vi "WebView_Init.vi"(8 "Error In":errorcluster, 11 "object in":refnum<class "WebView.lvclass">) -> (0 "Error Out":errorcluster, 3 "object out":refnum<class "WebView.lvclass">)   [LabVIEW 2024, in "WebView.lvclass"]
uses:
  WebView.lvclass
  WebView.lvclass/WebView.ctl
  <vilib>/sklein/WebView2/Libs/Microsoft.Web.WebView2.Core.dll
  Resources--cluster.ctl
  <vilib>/sklein/WebView2/Webview2 Control/Source Changed Event Data.ctl
  <vilib>/sklein/WebView2/Webview2 Control/WebView2 Control.xctl
  <vilib>/sklein/WebView2/Webview2 Control/Navigation Start Event Data.ctl
  <vilib>/sklein/WebView2/Webview2 Control/Navigation Event Data.ctl
  Events--cluster.ctl
  Navigation Event Data--cluster.ctl
  Source Changed Event Data--cluster.ctl
  Navigation Start Event Data--cluster.ctl
  <vilib>/sklein/WebView2/Libs/Microsoft.Web.WebView2.WinForms.dll
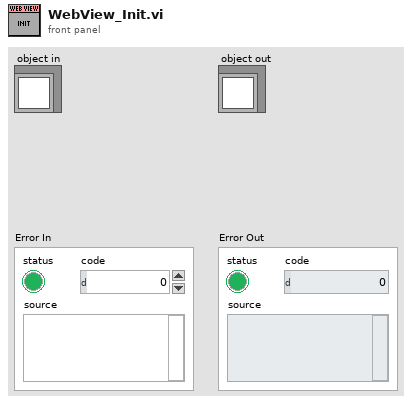
[diagram p1: front panel]
types:
  T1 = typedef "Navigation Start Event Data--cluster.ctl" = cluster{"AdditionalAllowedFrameAncestors":string, "Cancel":bool, "IsRedirected":bool, "IsUserInitiated":bool, "NavigationId":u64, "NavigationKind":i32, "RequestHeaders":refnum<k24>, "Uri":string}
  T2 = typedef "Navigation Event Data--cluster.ctl" = cluster{"HttpStatusCode":i32, "IsSuccess?":bool, "NavigationId":u64, "WebErrorStatus":i32}
  T3 = cluster{"Source":string, "WebMessageAsJson":string}
  T4 = typedef "WebView.lvclass/Events--cluster.ctl" = cluster{"Navigation Complete Event":refnum<user-event>, "Source Changed Event":refnum<user-event>, "Document Title Changed Event":refnum<user-event>, "Status Bar Text Changed":refnum<user-event>, "Web Message Received":refnum<user-event>, "Window Close Requested":refnum<user-event>, "DOM Loaded":refnum<user-event>, "Navigation Started Event":refnum<user-event>}
  T5 = typedef "Source Changed Event Data--cluster.ctl" = cluster{"Source":string, "IsNewDocument":bool}
  T6 = typedef "WebView.lvclass/Resources--cluster.ctl" = cluster{"WebView2":refnum<k24>, "Webview2 Core":refnum<k24>, "event callback":refnum<k27>, "Environment":refnum<k24>}
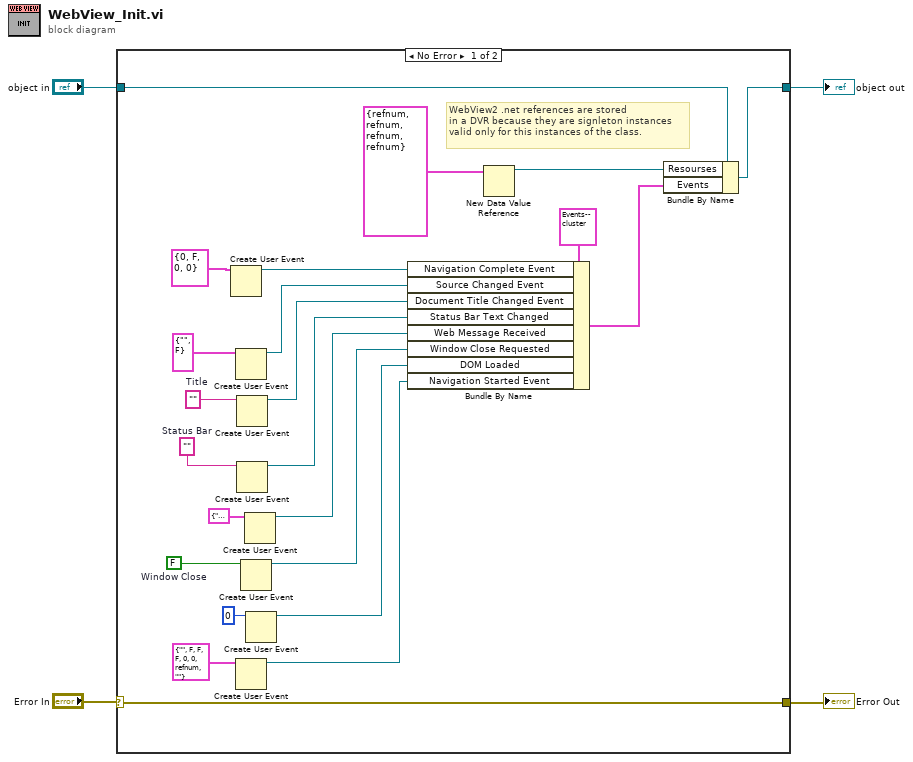
[diagram p0: block diagram]
diagram:
  n1 = case shown="No Error" "Error In" {
    selector: "Error In" -> [w27 w28]
    tunnel: "object in" -> [w25 w29]
    tunnel: [w26 w29] -> w3
    tunnel: [w27 w28] -> w1
    frame No Error {
      w13 = FALSE  # Window Close
      w16 = ""  # Status Bar
      w21 = ""  # Title
      # "WebView2 .net references are stored \nin a DVR because they are signleton instances\nvalid only for this instances of the class."
      n2 = Create User Event(user event datatype=T2 {"HttpStatusCode"=0, "IsSuccess?"=FALSE, "NavigationId"=0, "WebErrorStatus"=0} ("output cluster")) -> (user event=w18:refnum<user-event>)  [unwired: 1 in, 1 out]
      n3 = Create User Event(user event datatype=T5 {"Source"="", "IsNewDocument"=FALSE} ("Source")) -> (user event=w17:refnum<user-event>)  [unwired: 1 in, 1 out]
      n4 = Create User Event(user event datatype=T1 {"AdditionalAllowedFrameAncestors"="", "Cancel"=FALSE, "IsRedirected"=FALSE, "IsUserInitiated"=FALSE, "NavigationId"=0, "NavigationKind"=0, "RequestHeaders"=refnum, "Uri"=""} ("Nav Started Event")) -> (user event=w7:refnum<user-event>)  [unwired: 1 in, 1 out]
      n5 = Create User Event(user event datatype=w21) -> (user event=w19:refnum<user-event>)  [unwired: 1 in, 1 out]
      n6 = Create User Event(user event datatype=w16) -> (user event=w15:refnum<user-event>)  [unwired: 1 in, 1 out]
      n7 = Create User Event(user event datatype=w13) -> (user event=w12:refnum<user-event>)  [unwired: 1 in, 1 out]
      n8 = Create User Event(user event datatype=T3 {"Source"="", "WebMessageAsJson"=""} ("output cluster")) -> (user event=w14:refnum<user-event>)  [unwired: 1 in, 1 out]
      n9 = Create User Event(user event datatype=u64 0 ("NavigationId")) -> (user event=w10:refnum<user-event>)  [unwired: 1 in, 1 out]
      n10 = Bundle By Name(cluster=T4 {"Navigation Complete Event"=refnum, "Source Changed Event"=refnum, "Document Title Changed Event"=refnum, "Status Bar Text Changed"=refnum, "Web Message Received"=refnum, "Window Close Requested"=refnum, "DOM Loaded"=refnum, "Navigation Started Event"=refnum} ("Cluster"), "Navigation Complete Event"=w18, "Source Changed Event"=w17, "Document Title Changed Event"=w19, "Status Bar Text Changed"=w15, "Web Message Received"=w14, "Window Close Requested"=w12, "DOM Loaded"=w10, "Navigation Started Event"=w7) -> (w5:T4)
      n11 = New Data Value Reference(data value=T6 {"WebView2"=refnum, "Webview2 Core"=refnum, "event callback"=refnum, "Environment"=refnum}) -> (data value reference=w23:refnum<data-value>)  [unwired: 1 in, 1 out]
      n12 = Bundle By Name(cluster=w25, "Resourses"=w23, "Events"=w5) -> (w26:refnum<class "WebView.lvclass">)
    }
    frame Error {
    }
  }
  "object out" <- w3
  "Error Out" <- w1
